vi "changeState.vi"(8 "error in (no error)":errorcluster, 10 "State":refnum<class "State.lvclass">, 11 "Player in":refnum<class "Player.lvclass">) -> (0 "error out":errorcluster, 3 "Player out":refnum<class "Player.lvclass">)   [LabVIEW 2018, in "Player.lvclass"]
uses:
  Player.lvclass
  State Class/State.lvclass
  Player.lvclass/Player.ctl
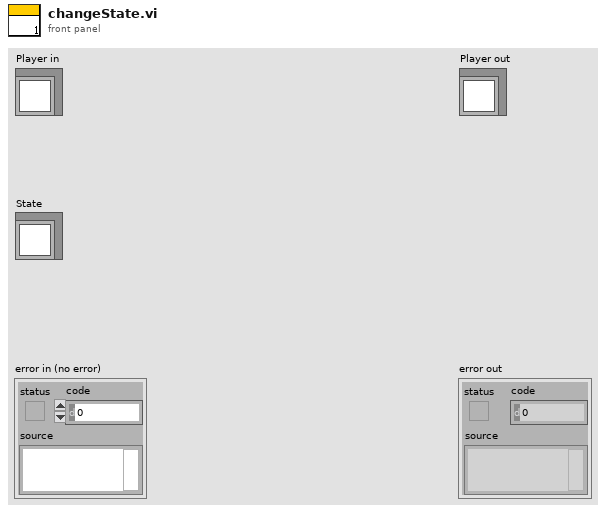
[diagram p1: front panel]
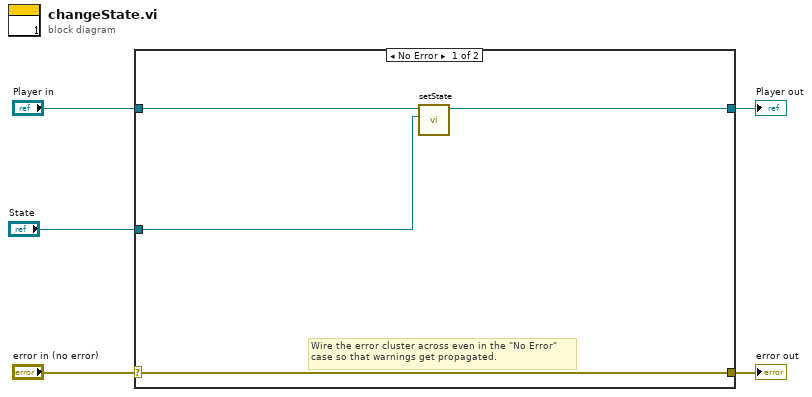
[diagram p0: block diagram]
diagram:
  n1 = case shown="No Error" "error in (no error)" {
    selector: "error in (no error)" -> [w8 w11]
    tunnel: [w8 w11] -> w4
    tunnel: [w7 w10] -> w2
    tunnel: "Player in" -> [w9 w10]
    tunnel: "State" -> [w6 _]
    frame No Error {
      # "Wire the error cluster across even in the \"No Error\"\ncase so that warnings get propagated."
      n2 = call "setState.vi"("State.lvclass"=w6, "Player in"=w9) -> ("Player out"=w7:refnum<class "Player.lvclass">)  [unwired: 8 in, 1 out]
    }
    frame Error {
    }
  }
  "error out" <- w4
  "Player out" <- w2
